vi "Get Position from String.vi"(11 "DataIn":string) -> (3 "Numeric":dbl)   [LabVIEW 2013, in "Airmar Data.lvclass"]
uses:
  Airmar Data.lvclass
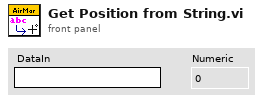
[diagram p1: front panel]
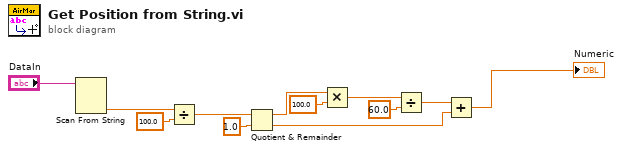
[diagram p0: block diagram]
diagram:
  n1 = Scan From String(input string="DataIn") -> (output 1=w2:dbl)  [unwired: 4 in, 3 out]
  n2 = Divide(x=w2, y=100.0) -> (x/y=w4:dbl)
  n3 = Quotient & Remainder(x=w4, y=1.0) -> (x-y*floor(x/y)=w8:dbl, floor(x/y)=w6:dbl)
  n4 = Multiply(x=w8, y=100.0) -> (x*y=w10:dbl)
  n5 = Divide(x=w10, y=60.0) -> (x/y=w12:dbl)
  n6 = Add(x=w12, y=w6) -> (x+y=→"Numeric":dbl)
